vi "State Machine Example.vi"   [LabVIEW 2017]
types:
  T1 = enum16{"Off", "Move Motor", "Wait", "Stop Motor"}
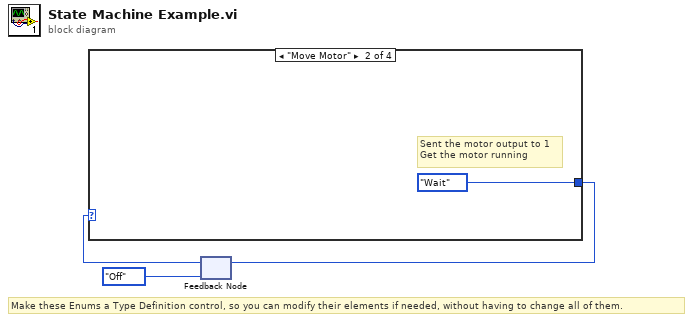
[diagram p0: block diagram]
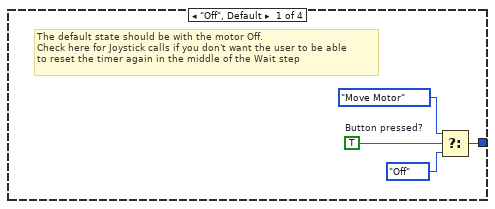
[diagram p2: hidden frame]
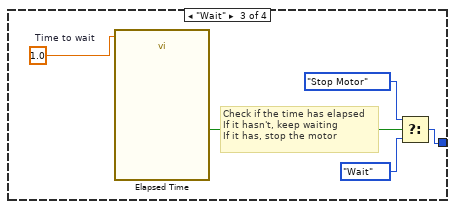
[diagram p3: hidden frame]
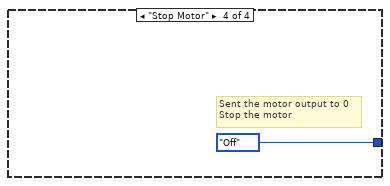
[diagram p4: hidden frame]
diagram:
  # "Make these Enums a Type Definition control, so you can modify their elements if needed, without having to change all of them."
  n1 = feedback #1(T1."Off") -> (w2:T1)
  n2 = case shown="\"Move Motor\"" w2 {
    tunnel: [w5 T1."Wait" w10 T1."Off"] -> w3
    frame "Off", Default {
      w4 = TRUE  # Button pressed?
      # "The default state should be with the motor Off. \nCheck here for Joystick calls if you don't want the user to be able\nto reset the timer again in the middle of the Wait step"
      n3 = Select(t=T1."Move Motor", s=w4, f=T1."Off") -> (s? t:f=w5:T1)
    }
    frame "Move Motor" {
      # "Sent the motor output to 1\nGet the motor running"
    }
    frame "Wait" {
      w13 = 1.0  # Time to wait
      # "Check if the time has elapsed\nIf it hasn't, keep waiting\nIf it has, stop the motor"
      n4 = call "Elapsed Time"("Time Target (s)"=w13) -> ("Time has Elapsed"=w9:bool)  [unwired: 11 in, 7 out]
      n5 = Select(t=T1."Stop Motor", s=w9, f=T1."Wait") -> (s? t:f=w10:T1)
    }
    frame "Stop Motor" {
      # "Sent the motor output to 0\nStop the motor"
    }
  }
  n6 = feedback-in #1(w3) -> ()
